vi "Update parameters (single).vi"(10 "New Parameter":cluster{"Name":string, "Value":string}, 11 "Parameters":cluster{"Name":string, "Value":string}[](array[cluster])) -> (3 "Parameters Out":cluster{"Name":string, "Value":string}[](array[cluster]))   [LabVIEW 2020, in "Measurement.lvclass"]
uses:
  Measurement.lvclass
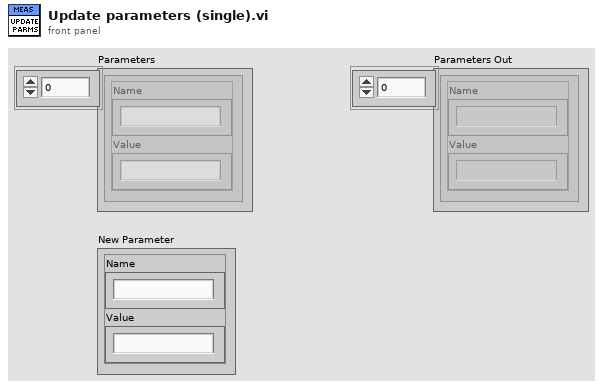
[diagram p1: front panel]
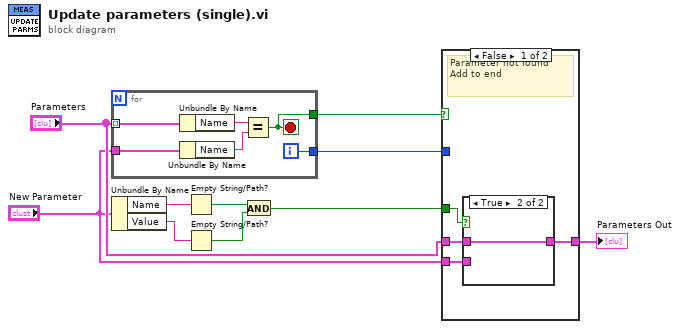
[diagram p0: block diagram]
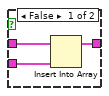
[diagram p2: hidden frame]
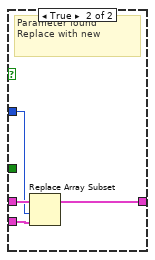
[diagram p3: hidden frame]
diagram:
  n1 = for {
    tunnel: "Parameters" -> [w16] mode=indexing
    tunnel: "New Parameter" -> [w15]
    tunnel: [w12] -> w10
    tunnel: [w11] -> w9
    i -> [w11]
    stop <- w12 stop-if-true
    n2 = Unbundle By Name(w16) -> ("Name"=w14:string)
    n3 = Unbundle By Name(w15) -> ("Name"=w13:string)
    n4 = Equal?(x=w14, y=w13) -> (x = y?=w12:bool)
  }
  n5 = Unbundle By Name("New Parameter") -> ("Name"=w5:string, "Value"=w4:string)
  n6 = Empty String/Path?(string/path=w5) -> (empty?=w3:bool)
  n7 = Empty String/Path?(string/path=w4) -> (empty?=w2:bool)
  n8 = And(x=w3, y=w2) -> (x .and. y?=w1:bool)
  n9 = case shown="False" w10 {
    tunnel: w9 -> [_ w27]
    tunnel: "Parameters" -> [w20 w28]
    tunnel: "New Parameter" -> [w18 w26]
    tunnel: [w19 w25] -> w7
    tunnel: w1 -> [w17 _]
    frame False {
      # "Parameter not found\nAdd to end"
      n10 = case shown="True" w17 {
        tunnel: w20 -> [w23 w24]
        tunnel: [w22 w24] -> w19
        tunnel: w18 -> [w21 _]
        frame False {
          n11 = Insert Into Array(array=w23, new element=w21) -> (w22:cluster{"Name":string, "Value":string}[])  [unwired: 1 in]
        }
        frame True {
        }
      }
    }
    frame True {
      # "Parameter found\nReplace with new"
      n12 = Replace Array Subset(array=w28, new element=w26, index=w27) -> (w25:cluster{"Name":string, "Value":string}[])
    }
  }
  "Parameters Out" <- w7
